vi "综合实验3.vi"() -> ()   [LabVIEW 2018]
uses:
  <vilib>/Analysis/2dsp.llb/Power Spectrum (DBL).vi
  <vilib>/Analysis/2dsp.llb/1D Auto Correlation (DBL).vi
  <vilib>/express/express analysis/Spectral/Block/exnSpectralBlock spectral measurements RMS poly.vi
  <vilib>/express/express analysis/Spectral/Block/exnSpectralBlock spectral measurements RMS WFM.vi
  <vilib>/express/express analysis/Spectral/XNode/ExpressSpectralMeasurementsBlockNode.xnode
  <vilib>/Analysis/NI_AALPro.lvlib
  <vilib>/measure/NI_MABase.lvlib
  <vilib>/measure/NI_MAPro.lvlib
panel:
  out "波峰因数":dbl format="%#_5g"
  in  "多频相位设置":dbl[](array[numeric])=[5.0, 4.0, 2.0, 3.0] format="%#_13g"
  in  "多频幅度设置":dbl[](array[numeric])=[4.0, 2.0, 4.0, 1.0] format="%#_13g"
  in  "多频频率设置":dbl[](array[numeric])=[4.0, 3.0, 4.0, 3.0] format="%#_13g"
  in  "振幅缩放设置":dbl=2.0 format="%#_13g"
  in  "公式":string="sin(w*t)*sin(2*pi(1)*t)\n\n"
  in  "噪声幅值":dbl(slide)=3.2323232323232323 scale=0.0..10.0
  out "功率谱":dbl[](graph)
  out "示波器":waveform(dbl)(graph)
  in  "采样信息":cluster{"数值":dbl, "数值 2":dbl}={"数值"=200.0, "数值 2"=200.0}
  in  "方波占空比 2":dbl(knob)=8.501312514606928 scale=0.0..10.0
  out "相位 2":dbl format="%#_13g"
  in  "相位":dbl(knob)=5.040052625582293 scale=0.0..10.0
  out "幅度 2":dbl format="%#_13g"
  in  "幅度":dbl(knob)=2.96571345613434 scale=0.0..10.0
  out "频率 2":dbl format="%#_13g"
  in  "频率":dbl(knob)=5.255989724503292 scale=0.0..10.0
  out "偏移量 2":dbl format="%#_13g"
  in  "signal type":T1(ring) caption="信号类型"
  out "方波占空比":dbl format="%#_13g"
  in  "偏移量":dbl(knob)=5.595635015377106 scale=0.0..10.0
  out "自相关":dbl[](graph)
  out "积分":dynamicdata(graph)
  out "微分":dynamicdata(graph)
  out "频谱分析":cluster{"f0":dbl, "df":dbl, "magnitude":dbl[]}(graph)
  in  "停止":bool
  in  "波形选择":enum16{"常见波形", "噪声波形", "公式波形", "多频波形"}(ring)
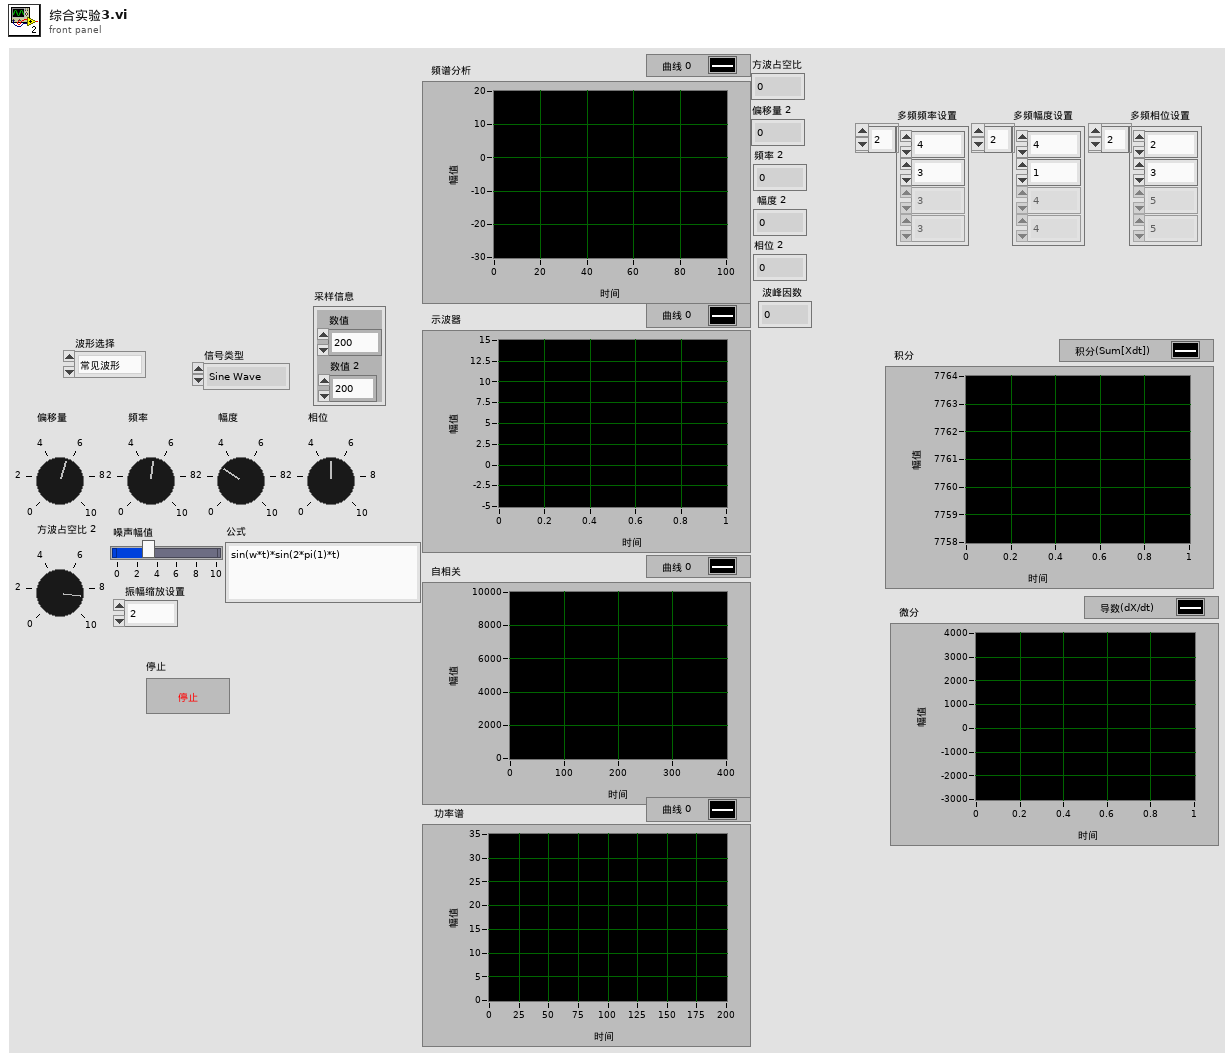
[diagram p1: front panel]
types:
  T1 = enum16{"Sine Wave", "Triangle Wave", "Square Wave", "Sawtooth Wave"}
  T2 = cluster{"averaging mode":u16, "weighting mode":u16, "number of averages":u32}
  T3 = cluster{"dB On (F)":bool, "unwrap phase (F)":bool, "convert to degree (F)":bool}
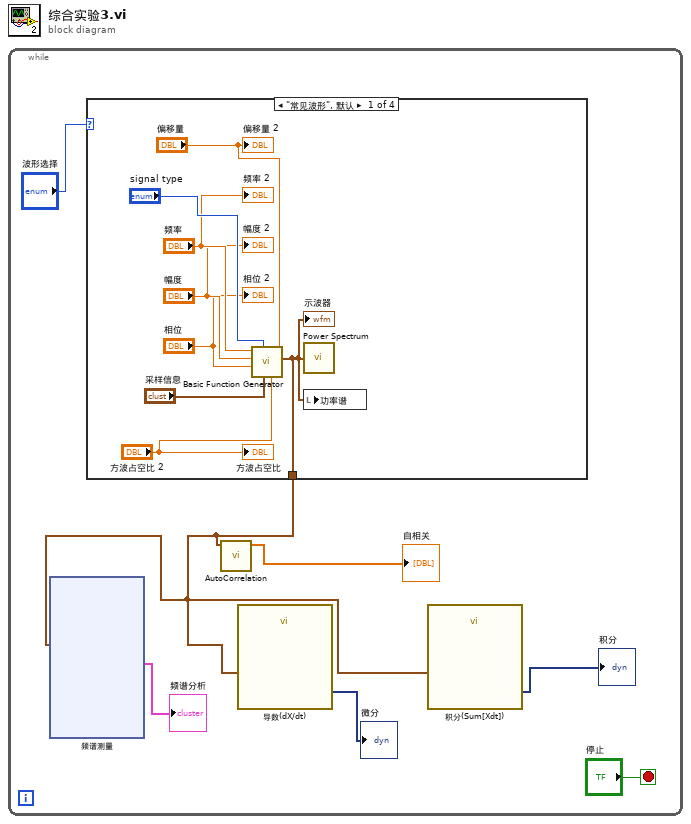
[diagram p0: block diagram]
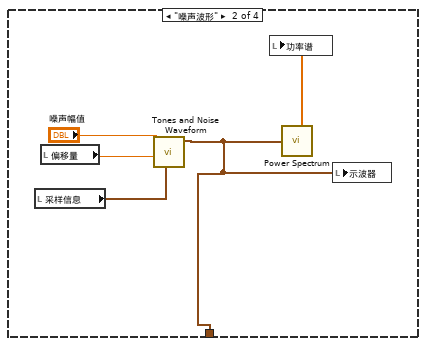
[diagram p2: hidden frame]
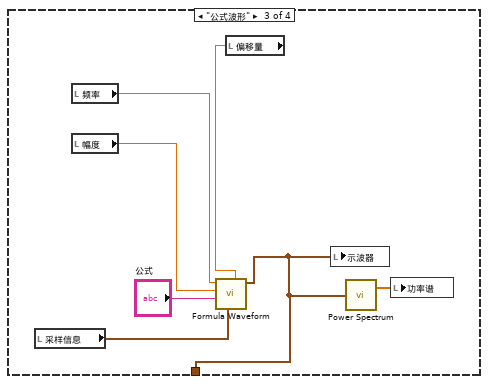
[diagram p3: hidden frame]
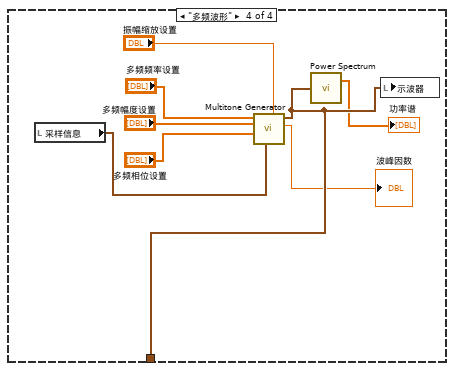
[diagram p4: hidden frame]
diagram:
  n1 = while {
    stop <- "停止" stop-if-true
    n2 = case shown="\"常见波形\", 默认" "波形选择" {
      tunnel: [w8 w16 w26 w30] -> w1
      frame "常见波形", Default {
        n3 = call <vilib>:"Basic Function Generator.vi"("offset"="偏移量", "square wave duty cycle (%)"="方波占空比 2", "sampling info"="采样信息", "signal type"="signal type", "phase"="相位", "amplitude"="幅度", "frequency"="频率") -> ("signal out"=w8:waveform(dbl))  [unwired: 2 in, 2 out]
        "示波器" <- w8
        n4 = call-poly <vilib>:"Power Spectrum.vi"("X"=w8) -> ()  [unwired: 2 out]
        n5 = local write "功率谱"(w8) -> ()
        "方波占空比" <- "方波占空比 2"
        "偏移量 2" <- "偏移量"
        "频率 2" <- "频率"
        "幅度 2" <- "幅度"
        "相位 2" <- "相位"
      }
      frame "噪声波形" {
        n6 = local read "采样信息"() -> (w20:cluster{"数值":dbl, "数值 2":dbl})
        n7 = local read "偏移量"() -> (w17:dbl)
        n8 = call <vilib>:"Tones and Noise Waveform.vi"("sampling info"=w20, "offset"=w17, "noise (rms)"="噪声幅值") -> ("signal out"=w16:waveform(dbl))  [unwired: 7 in, 1 out]
        n9 = call-poly <vilib>:"Power Spectrum.vi"("X"=w16) -> ("Power Spectrum"=w19:dbl[])  [unwired: 1 out]
        n10 = local write "功率谱"(w19) -> ()
        n11 = local write "示波器"(w16) -> ()
      }
      frame "公式波形" {
        n12 = local read "采样信息"() -> (w24:cluster{"数值":dbl, "数值 2":dbl})
        n13 = local read "频率"() -> (w22:dbl)
        n14 = local read "幅度"() -> (w21:dbl)
        n15 = local read "偏移量"() -> (w23:dbl)
        n16 = call <vilib>:"Formula Waveform.vi"("offset"=w23, "sampling info"=w24, "formula"="公式", "amplitude"=w21, "frequency"=w22) -> ("signal out"=w26:waveform(dbl))  [unwired: 5 in, 1 out]
        n17 = local write "示波器"(w26) -> ()
        n18 = call-poly <vilib>:"Power Spectrum.vi"("X"=w26) -> ("Power Spectrum"=w27:dbl[])  [unwired: 1 out]
        n19 = local write "功率谱"(w27) -> ()
      }
      frame "多频波形" {
        n20 = local read "采样信息"() -> (w35:cluster{"数值":dbl, "数值 2":dbl})
        n21 = call <vilib>:"Multitone Generator.vi"("amplitude"="振幅缩放设置", "sampling info"=w35, "tone phases"="多频相位设置", "tone amplitudes"="多频幅度设置", "tone frequencies"="多频频率设置") -> ("crest factor"=→"波峰因数":dbl, "signal out"=w30:waveform(dbl))  [unwired: 3 in, 2 out]
        n22 = call-poly <vilib>:"Power Spectrum.vi"("X"=w30) -> ("Power Spectrum"=→"功率谱":dbl[])  [unwired: 1 out]
        n23 = local write "示波器"(w30) -> ()
      }
    }
    n24 = xnode "频谱测量"("信号"=w1) -> ("测量输出"=→"频谱分析":cluster{"f0":dbl, "df":dbl, "magnitude":dbl[]})  [unwired: 1 in, 2 out]
    n25 = call-poly <vilib>:"AutoCorrelation.vi"("X"=w1) -> ("Rxx"=→"自相关":dbl[])  [unwired: 9 in, 1 out]
    n26 = call "导数(dX/dt)"("Signals"=w1) -> ("Result"=→"微分":dynamicdata)  [unwired: 5 in, 1 out]
    n27 = call "积分(Sum[Xdt])"("Signals"=w1) -> ("Result"=→"积分":dynamicdata)  [unwired: 5 in, 1 out]
  }
